vi "testTrue.vi"(8 "error in (no error)":errorcluster) -> (0 "error out":errorcluster)   [LabVIEW 2019, in "AssertionTest.lvlib" / "AssertTrue.lvlib"]
uses:
  AssertTrue.lvlib
  Assertion/Assertion.lvlib
  AssertionTest.lvlib
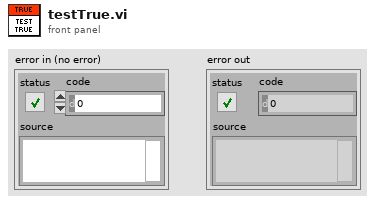
[diagram p1: front panel]
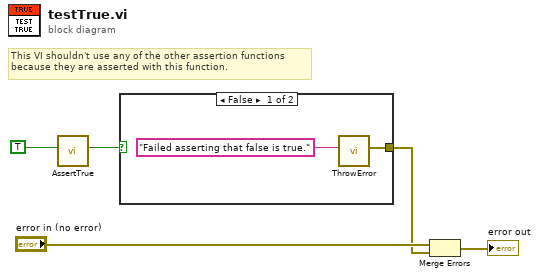
[diagram p0: block diagram]
diagram:
  # "This VI shouldn't use any of the other assertion functions\nbecause they are asserted with this function."
  n1 = call "AssertTrue.vi"("Condition"=TRUE) -> ("Result"=w4:bool)  [unwired: 9 in, 1 out]
  n2 = case shown="False" w4 {
    tunnel: [w6 _] -> w1
    frame False {
      n3 = call "ThrowError.vi"("Error Message"="Failed asserting that false is true." ("message")) -> ("error out"=w6:errorcluster)  [unwired: 10 in]
    }
    frame True {
    }
  }
  n4 = Merge Errors("error in (no error)", w1) -> (→"error out":errorcluster)
